vi "KE2260B Special Write.vi"(8 "error in (no error)":errorcluster, 10 "Write Buffer (\"\")":string, 11 "VISA session":refnum<visa-resource-name>) -> (0 "error out":errorcluster, 2 "Return Count":u32, 3 "dup VISA session":refnum<visa-resource-name>)   [LabVIEW 2009, in "Keithley 2260B.lvlib"]
doc: "RS232 message terminators: AS there is no signal of end message on RS232 bus, therefore, use LF as \nmessage terminator. When a series of commands are sent to the instrument, it must add a LF to be a\njudhment for message terminator. As for query command, the return message of the instrument is also\nadded a LF for PC to judge message terminator."
uses:
  <instrlib>/Keithley 2260B/Keithley 2260B.lvlib
panel:
  # "WARNINGS: \nRS232 message terminators: AS there is no signal of end message on RS232\nbus, therefore, use LF as message terminator. When a series of commands \nare sent to the instrument, it must add a LF to be a judhment for message\nterminator. As for query command, the return message of the instrument is\nalso added a LF for PC to judge message terminator."
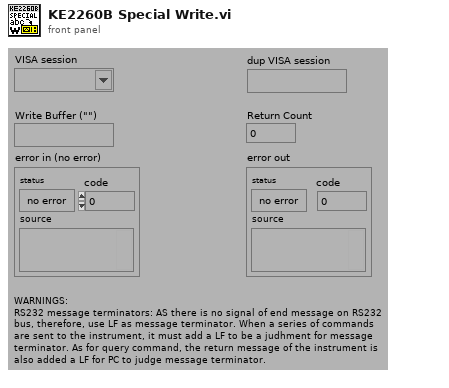
[diagram p1: front panel]
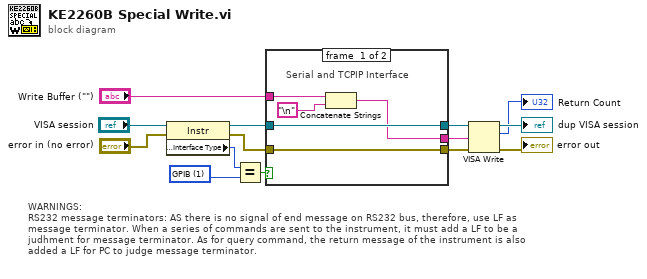
[diagram p0: block diagram]
diagram:
  w8 = u16 1 items=["GPIB"=1, "VXI"=2, "GPIB-VXI"=3, "Serial"=4, "PXI"=5] ("Interface Information:Interface Type")
  # "WARNINGS: \nRS232 message terminators: AS there is no signal of end message on RS232 bus, therefore, use LF as \nmessage terminator. When a series of commands are sent to the instrument, it must add a LF to be a\njudhment for message terminator. As for query command, the return message of the instrument is also\nadded a LF for PC to judge message terminator."
  n1 = property class="Instr"(reference="VISA session", error in="error in (no error)") -> (reference out=w10:refnum<visa-resource-name>, error out=w13:errorcluster, "Interface Information:Interface Type"=w7:u16)
  n2 = Equal?(x=w7, y=w8) -> (x = y?=w11:bool)
  n3 = case shown="False" w11 {
    tunnel: w13 -> [w17 w22]
    tunnel: w10 -> [w18 w21]
    tunnel: "Write Buffer (\"\")" -> [w19 w20]
    tunnel: [w18 w21] -> w6
    tunnel: [w17 w22] -> w5
    tunnel: [w16 w20] -> w2
    frame #0 {
      # "Serial and TCPIP Interface"
      n4 = Concatenate Strings(w19, "\n") -> (w16:string)
    }
    frame #1 {
      # "GPIB Interface"
    }
  }
  n5 = VISA Write(VISA resource name=w6, write buffer=w2, error in (no error)=w5) -> (VISA resource name out=→"dup VISA session":refnum<visa-resource-name>, return count=→"Return Count":u32, error out=→"error out":errorcluster)
